vi "ULS PMT.vi"(8 "error in (no error)":errorcluster, 10 "Dwell(ms)":dbl, 11 "IFD in":refnum<class "IFD.lvclass">) -> (0 "error out":errorcluster, 3 "IFD out":refnum<class "IFD.lvclass">)   [LabVIEW 2016, in "IFD.lvclass"]
uses:
  IFD.lvclass
  Tag/IFD_Tag.lvclass/IFD_Tag.ctl
  IFD.lvclass/IFD.ctl
  Tag/IFD_Tag.lvclass
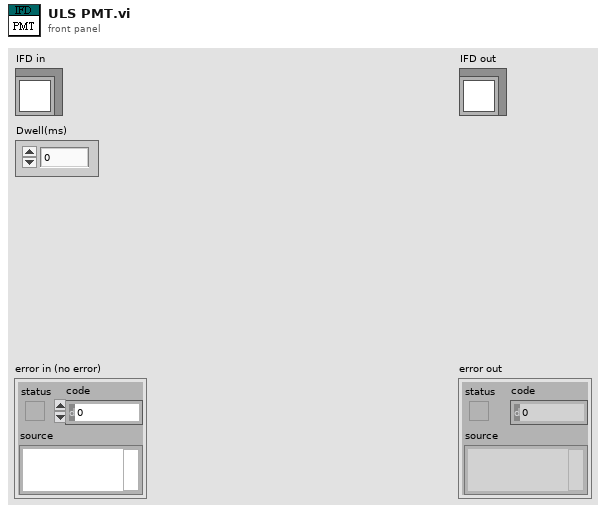
[diagram p1: front panel]
types:
  T1 = enum16{"Undefined(DO NOT USE)", "U8", "ASCII", "U16", "U32", "RATIONAL", "I8", "Undefined 8 bit", "I16", "I32", "SRATIONAL", "SGL", "DBL"}
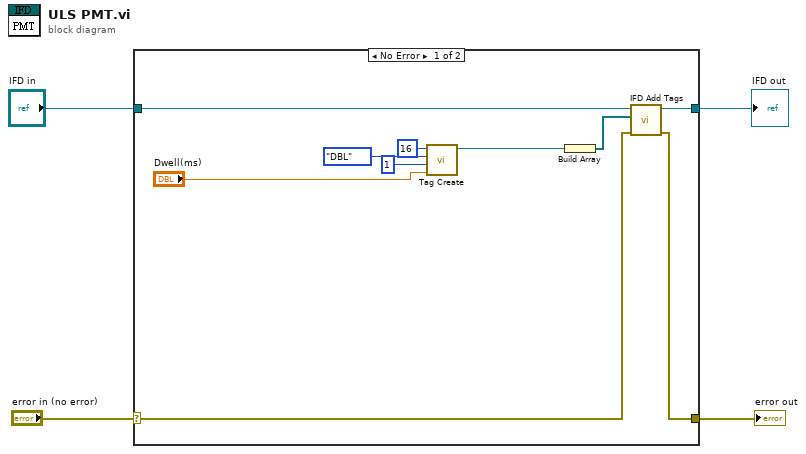
[diagram p0: block diagram]
diagram:
  n1 = case shown="No Error" "error in (no error)" {
    selector: "error in (no error)" -> [w14 w16]
    tunnel: [w13 w16] -> w3
    tunnel: [w12 w15] -> w1
    tunnel: "IFD in" -> [w11 w15]
    frame No Error {
      n2 = call "Tag Create.vi"("Data"="Dwell(ms)", "Data Count"=u32 1, "Data Type"=T1."DBL", "Tag ID"=u16 16) -> ("IFD_Tag out"=w5:refnum<class "IFD_Tag.lvclass">)  [unwired: 7 in]
      n3 = Build Array(w5) -> (w6:refnum<class "IFD_Tag.lvclass">[])
      n4 = call "IFD Add Tags.vi"("error in (no error)"=w14, "Tag(s)"=w6, "IFD in"=w11) -> ("error out"=w13:errorcluster, "IFD out"=w12:refnum<class "IFD.lvclass">)  [unwired: 7 in]
    }
    frame Error {
    }
  }
  "error out" <- w3
  "IFD out" <- w1
